vi "Register Groups.vi"(8 "error in (no error)":errorcluster, 9 "Promise":refnum<class "Promise.lvclass">, 10 "Groups":refnum<class "Group.lvclass">[](array[class]), 11 "DataLogger in":refnum<class "DataLogger.lvclass">) -> (0 "error out":errorcluster, 3 "DataLogger out":refnum<class "DataLogger.lvclass">)   [LabVIEW 2020, in "VolatusDataLogger.lvlib" / "DataLogger.lvclass"]
uses:
  DataLogger.lvclass
  DataLogger.lvclass/DataLogger.ctl
  lv-vecto/Vecto/GroupAbstract/GroupAbstract.lvclass
  lv-vecto/Vecto/Group Config/Group Config.lvclass
  lv-promises/Promises/Error Result/Error Result.lvclass
  lv-promises/Promises/Promise/Promise.lvclass
  lv-vecto/Vecto/Group/Group.lvclass
  C:/dev/lv20CE/relink/lv-vecto/Vecto/GroupAbstract/GroupAbstract.lvclass
  C:/dev/lv20CE/relink/lv-vecto/Vecto/Group/Group.lvclass
  C:/dev/lv20CE/relink/lv-promises/Promises/Value/Value.lvclass
  C:/dev/lv20CE/relink/lv-promises/Promises/Error Result/Error Result.lvclass
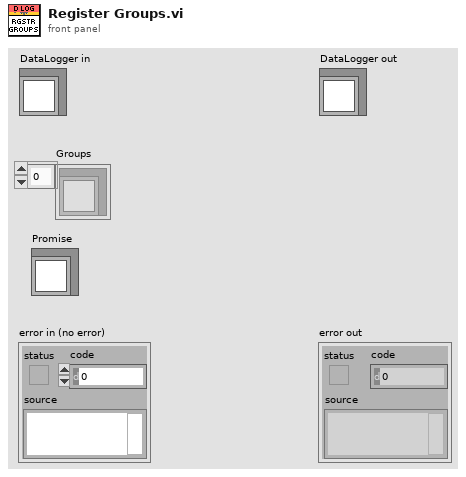
[diagram p1: front panel]
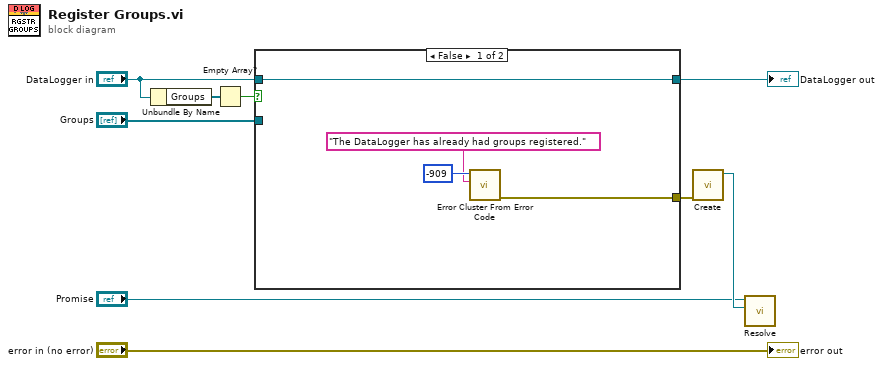
[diagram p0: block diagram]
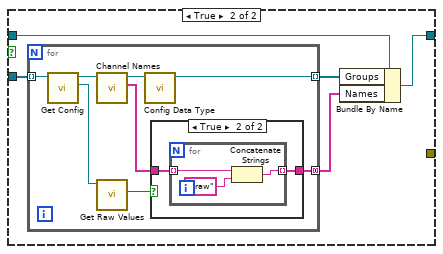
[diagram p2: hidden frame]
diagram:
  n1 = Unbundle By Name("DataLogger in") -> ("Groups"=w5:refnum<class "Group.lvclass">[])
  n2 = Empty Array?(array=w5) -> (empty?=w1:bool)
  n3 = case shown="False" w1 {
    tunnel: "Groups" -> [_ w18]
    tunnel: [w13 w17] -> w7
    tunnel: "DataLogger in" -> [w13 w14]
    tunnel: [w10 _] -> w4
    frame False {
      n4 = call <vilib>:"Error Cluster From Error Code.vi"("error message (\"\")"="The DataLogger has already had groups registered.", "error code (0)"=-909) -> ("error out"=w10:errorcluster)  [unwired: 7 in]
    }
    frame True {
      n5 = for {
        tunnel: w18 -> [w26] mode=indexing
        tunnel: [w19] -> w16 mode=indexing
        tunnel: [w20] -> w15 mode=concatenating
        n6 = call "Get Config.vi"("GroupAbstract in"=w26) -> ("Config"=w24:refnum<class "Group Config.lvclass">, "GroupAbstract out"=w25:refnum<class "Group.lvclass">)  [unwired: 8 in, 1 out]
        n7 = call "Channel Names.vi"("GroupAbstract in"=w25) -> ("Channel Names"=w21:string[], "GroupAbstract out"=w23:refnum<class "Group.lvclass">)  [unwired: 8 in, 1 out]
        n8 = call "Get Raw Values.vi"("Group Config in"=w24) -> ("Raw Values"=w22:bool)  [unwired: 8 in, 2 out]
        n9 = call "Config Data Type.vi"("GroupAbstract in"=w23) -> ("GroupAbstract out"=w19:refnum<class "Group.lvclass">)  [unwired: 8 in, 2 out]
        n10 = case shown="True" w22 {
          tunnel: w21 -> [w27 w29]
          tunnel: [w27 w28] -> w20
          frame False {
          }
          frame True {
            n11 = for {
              tunnel: w29 -> [w32] mode=indexing
              tunnel: [w30] -> w28 mode=indexing
              n12 = Concatenate Strings(w32, "_raw" ("string")) -> (w30:string)
            }
          }
        }
      }
      n13 = Bundle By Name(cluster=w14, "Groups"=w16, "Names"=w15) -> (w17:refnum<class "DataLogger.lvclass">)
    }
  }
  "DataLogger out" <- w7
  n14 = call "Create.vi"("error in (no error)"=w4) -> ("Error Result out"=w3:refnum<class "Error Result.lvclass">)  [unwired: 9 in, 1 out]
  n15 = call "Resolve.vi"("Result"=w3, "Promise in"="Promise") -> ()  [unwired: 8 in, 2 out]
  "error out" <- "error in (no error)"
